vi "CryoCon Load Calibration.vi"(0 "Instrument Address":refnum<visa-resource-name>, 1 "Sensor Type":T1=enum."AC Resistance", 2 "Sensor Number":u32=1 min=1 max=12 step=1, 3 "Error In":errorcluster, 4 "Calibration (Empty gives dialog)":string) -> (5 "dup VISA session":refnum<visa-resource-name>, 6 "Sensor ID":string, 8 "error out":errorcluster {"code" format="%.0x"})   [LabVIEW 2025]
doc: "This VI loads a calibration file into the Conductus LTC-20 temperature controller. The file is a line of up to 19 characters of ID info, followed by the temperature information in 2 columns of temperature and resistance (sensor value)\nScott Hannahs, NHMFL-FSU, March 1995\nAuthor: Scott Hannahs <sth@magnet.fsu.edu>\n\nThis software is licensed for use under the “MIT License\"\nCopyright (c) 2025 Scott Hannahs, sth@sth@magnet.sthnet.net\n\nPermission is hereby granted, free of charge, to any person obtaining a copy of this software and associated documentation files (the \"Software\"), to deal in the Software without restriction, including without limitation the rights to use, copy, modify, merge, publish, distribute, sublicense, and/or sell copies of the Software, and to permit persons to whom the Software is furnished to do so, subject to the following conditions: The above copyright notice and this permission notice shall be included in all copies or substantial portions of the Software.\n\nTHE SOFTWARE IS PROVIDED \"AS IS\", WITHOUT WARRANTY OF ANY KIND, EXPRESS OR IMPLIED, INCLUDING BUT NOT LIMITED TO THE WARRANTIES OF MERCHANTABILITY, FITNESS FOR A PARTICULAR PURPOSE AND NONINFRINGEMENT. IN NO EVENT SHALL THE AUTHORS OR COPYRIGHT HOLDERS BE LIABLE FOR ANY CLAIM, DAMAGES OR OTHER LIABILITY, WHETHER IN AN ACTION OF CONTRACT, TORT OR OTHERWISE, ARISING FROM, OUT OF OR IN CONNECTION WITH THE SOFTWARE OR THE USE OR OTHER DEALINGS IN THE SOFTWARE."
uses:
  Sub Controls/CryoCon Sensor Type.ctl
  <vilib>/Utility/error.llb/Trim Whitespace One-Sided.vi
panel:
  out "Status":string
  out "String Read":string
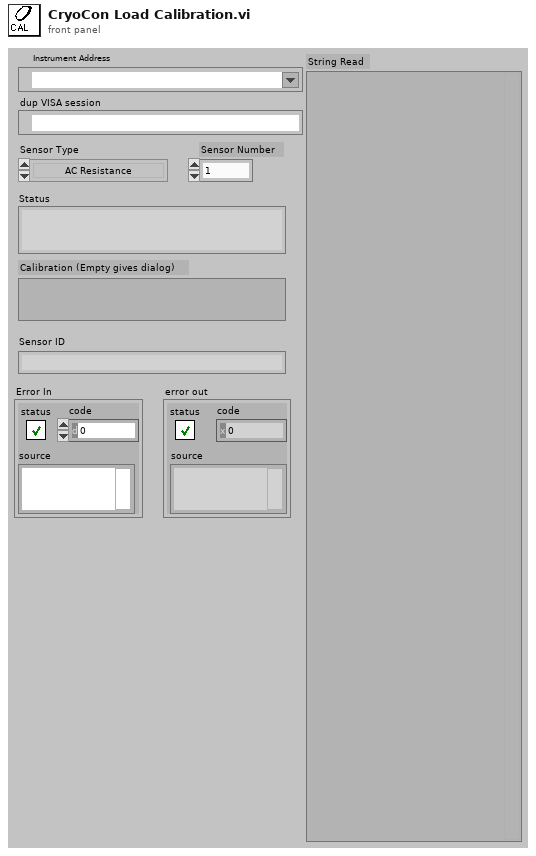
[diagram p1: front panel]
types:
  T1 = typedef "CryoCon Sensor Type.ctl" = enum16{"Diode", "AC Resistance", "DC Resistance 3.1 k½", "DC Resistance 312 ½", "DC Resistance 625 ½"}
  T2 = enum32{"Invalid", "Standard", "Closed", "Hidden", "Minimized", "Maximized"}
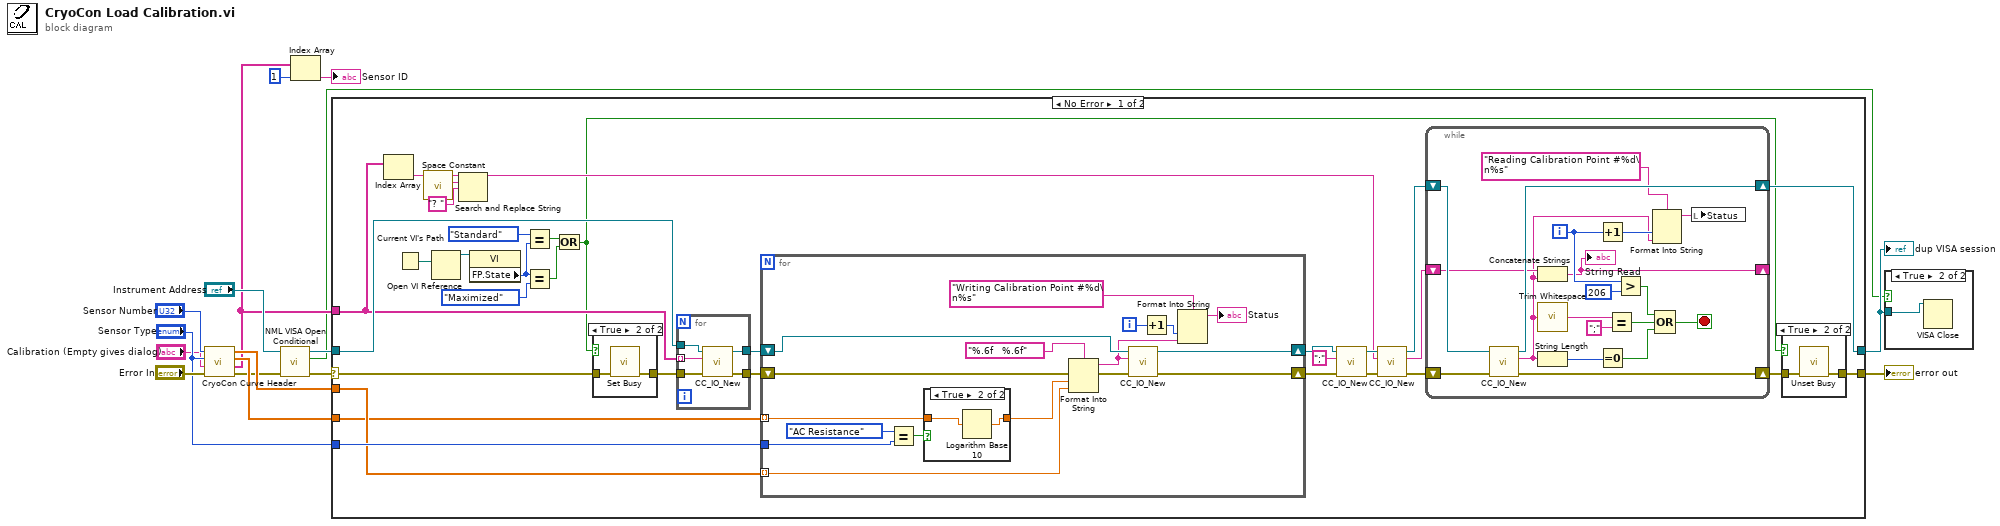
[diagram p0: block diagram]
diagram:
  n1 = call "CryoCon Curve Header.vi"("Error In"="Error In", "Calibration (Empty gives dialog)"="Calibration (Empty gives dialog)", "Sensor Type"="Sensor Type", "Sensor Number"="Sensor Number") -> ("error out"=w2:errorcluster, "Header Array"=w6:string[], "Resistance"=w13:dbl[], "Temperature"=w14:dbl[])
  n2 = call "NML VISA Open Conditional.vi"("error in (no error)"=w2, "VISA resource name"="Instrument Address") -> ("error out"=w1:errorcluster, "Opened?"=w3:bool, "dup VISA Session"=w4:refnum<visa-resource-name>)  [unwired: 7 in]
  n3 = Index Array(array=w6, index=1) -> (element=→"Sensor ID":string)
  n4 = case shown="No Error" w1 {
    selector: w1 -> [w38 w99]
    tunnel: w6 -> [w36 _]
    tunnel: "Sensor Type" -> [w48 _]
    tunnel: [w37 w99] -> w15
    tunnel: [w27 w100] -> w10
    tunnel: w14 -> [w44 _]
    tunnel: w13 -> [w43 _]
    tunnel: w4 -> [w40 w100]
    frame No Error {
      n5 = Index Array(array=w36) -> (element=w25:string)  [unwired: 1 in]
      n6 = Current VI's Path() -> (path=w18:path)
      n7 = call <vilib>:"Space Constant.vi"() -> ("String"=w32:string)
      n8 = Open VI Reference(vi path=w18) -> (vi reference=w24:refnum<vi>)  [unwired: 5 in, 1 out]
      n9 = Search and Replace String(input string=w25, search string=w32, replace string="? " ("replace string (\"\")")) -> (result string=w33:string)  [unwired: 5 in, 3 out]
      n10 = property class="VI"(reference=w24) -> ("FP.State"=w21:T2)  [unwired: 1 in, 2 out]
      n11 = Equal?(x=T2."Standard" ("Front Panel Window:State"), y=w21) -> (x = y?=w20:bool)
      n12 = Equal?(x=w21, y=T2."Maximized" ("Front Panel Window:State")) -> (x = y?=w19:bool)
      n13 = Or(x=w20, y=w19) -> (x .or. y?=w17:bool)
      n14 = case shown="True" w17 {
        tunnel: [w52 w54] -> w39
        tunnel: w38 -> [w52 w53]
        frame False {
        }
        frame True {
          n15 = call <vilib>:"Set Busy.vi"("error in (no error)"=w53) -> ("error out"=w54:errorcluster)  [unwired: 9 in, 1 out]
        }
      }
      n16 = for {
        tunnel: w36 -> [w74] mode=indexing
        tunnel: w39 -> [w78]
        tunnel: [w77] -> w47
        tunnel: [w76] -> w45
        tunnel: w40 -> [w75]
        n17 = call "CC_IO_New.vi"("error in (no error)"=w78, "Command String"=w74, "VISA Refnum in"=w75) -> ("error out"=w77:errorcluster, "VISA Refnum out"=w76:refnum<visa-resource-name>)  [unwired: 6 in, 1 out]
      }
      n18 = for {
        tunnel: w48 -> [w95]
        shift-right: [w91] -> w41
        shift-left: w47 -> [w93]
        shift-right: [w92] -> w42
        shift-left: w45 -> [w90]
        tunnel: w44 -> [w85] mode=indexing
        tunnel: w43 -> [w87] mode=indexing
        i -> [w83]
        n19 = Equal?(x=CryoCon_Sensor_Type."AC Resistance" ("Sensor Type"), y=w95) -> (x = y?=w94:bool)
        n20 = case shown="True" w94 {
          tunnel: w87 -> [w96 w98]
          tunnel: [w96 w97] -> w84
          frame False {
          }
          frame True {
            n21 = Logarithm Base 10(1:w98) -> (0:w97:dbl)
          }
        }
        n22 = Format Into String(format string="%.6f   %.6f" ("Format String"), error in=w93, w84, w85) -> (resulting string=w79:string, error out=w88:errorcluster)  [unwired: 1 in]
        n23 = call "CC_IO_New.vi"("error in (no error)"=w88, "Command String"=w79, "VISA Refnum in"=w90) -> ("error out"=w91:errorcluster, "VISA Refnum out"=w92:refnum<visa-resource-name>)  [unwired: 6 in, 1 out]
        n24 = Increment(x=w83) -> (x+1=w82:i32)
        n25 = Format Into String(format string="Writing Calibration Point #%d\n%s", w82, w79) -> (resulting string=→"Status":string)  [unwired: 2 in, 1 out]
      }
      n26 = call "CC_IO_New.vi"("error in (no error)"=w41, "Command String"=";", "VISA Refnum in"=w42) -> ("error out"=w34:errorcluster, "VISA Refnum out"=w35:refnum<visa-resource-name>)  [unwired: 6 in, 1 out]
      n27 = call "CC_IO_New.vi"("error in (no error)"=w34, "Command String"=w33, "VISA Refnum in"=w35) -> ("error out"=w30:errorcluster, "String Read"=w26:string, "VISA Refnum out"=w28:refnum<visa-resource-name>)  [unwired: 6 in]
      n28 = while {
        shift-right: [w57] -> _
        shift-left: w26 -> [w69]
        shift-right: [w72] -> w29
        shift-left: w30 -> [w73]
        shift-right: [w70] -> w27
        shift-left: w28 -> [w71]
        i -> [w62]
        stop <- w65 stop-if-true
        n29 = call "CC_IO_New.vi"("error in (no error)"=w73, "VISA Refnum in"=w71) -> ("error out"=w72:errorcluster, "String Read"=w55:string, "VISA Refnum out"=w70:refnum<visa-resource-name>)  [unwired: 7 in]
        n30 = Concatenate Strings(w69, w55) -> (w57:string)
        "String Read" <- w57
        n31 = call <vilib>:"Trim Whitespace.vi"("string"=w55) -> ("trimmed string"=w56:string)  [unwired: 1 in]
        n32 = String Length(string=w55) -> (length=w59:i32)
        n33 = Increment(x=w62) -> (x+1=w64:i32)
        n34 = Equal To 0?(x=w59) -> (x = 0?=w58:bool)
        n35 = Equal?(x=w56, y=";") -> (x = y?=w66:bool)
        n36 = Greater?(x=w62, y=206) -> (0:w60:bool)
        n37 = Format Into String(format string="Reading Calibration Point #%d\n%s", w64, w55) -> (resulting string=w61:string)  [unwired: 2 in, 1 out]
        n38 = Compound Arithmetic op=OR(w60, w66, w58) -> (w65:bool)
        n39 = local write "Status"(w61) -> ()
      }
      n40 = case shown="True" w17 {
        tunnel: [w49 w51] -> w37
        tunnel: w29 -> [w49 w50]
        frame False {
        }
        frame True {
          n41 = call <vilib>:"Unset Busy.vi"("error in (no error)"=w50) -> ("error out"=w51:errorcluster)  [unwired: 10 in]
        }
      }
    }
    frame Error {
    }
  }
  "dup VISA session" <- w10
  "error out" <- w15
  n42 = case shown="True" w3 {
    tunnel: w10 -> [_ w101]
    frame False {
    }
    frame True {
      n43 = VISA Close(VISA resource name=w101) -> ()  [unwired: 1 in, 1 out]
    }
  }
